vi "Connect.vi"(8 "error in (no error)":errorcluster, 9 "timeout":i32=-1, 11 "Message Stream in":refnum<class "Message Stream.lvclass">) -> (0 "error out":errorcluster, 3 "Message Stream out":refnum<class "Message Stream.lvclass">)   [LabVIEW 2020, in "Message Stream.lvclass"]
doc: "Override this method to specify the action the local copy of this object will perform to connect to its remote counterpart."
uses:
  Message Stream.lvclass
  <vilib>/Utility/error.llb/Error Cluster From Error Code.vi
  <vilib>/ErrorRing/Error Ring.xnode
  Message Stream.lvclass/Message Stream.ctl
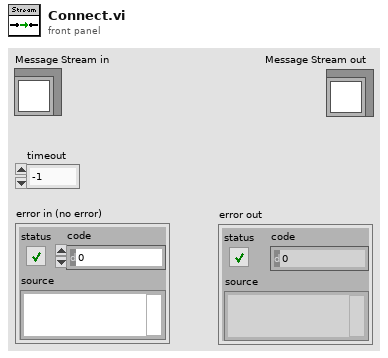
[diagram p1: front panel]
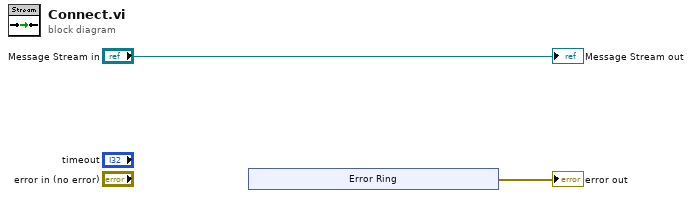
[diagram p0: block diagram]
diagram:
  n1 = xnode "Error Ring"() -> ("error out"=→"error out":errorcluster)
  "Message Stream out" <- "Message Stream in"
